vi "IMU Correction.vi"(9 "Heading Setpoint":dbl, 10 "theta":dbl) -> (3 "Difference":dbl)   [LabVIEW 2020]
panel:
  out "IMU Correction":T1(graph)
  in  "PID gains":T2={"proportional gain (Kp)"=4.0, "integral time (Ki)"=0.0, "derivative time (Kd)"=0.0} {"derivative time (Kd)" format="%.3f"; "integral time (Ki)" format="%.3f"; "proportional gain (Kp)" format="%.3f"}
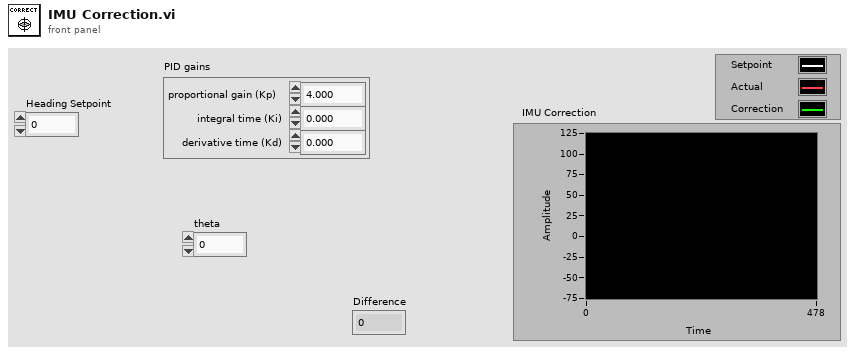
[diagram p1: front panel]
types:
  T1 = cluster{"Heading Setpoint":dbl, dbl, "output":dbl}
  T2 = cluster{"proportional gain (Kp)":dbl, "integral time (Ki)":dbl, "derivative time (Kd)":dbl}
  T3 = cluster{"Heading Setpoint":dbl, "theta":dbl, "output":dbl}
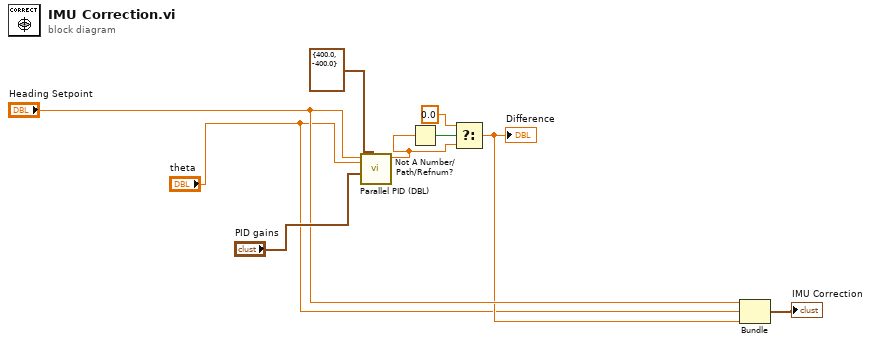
[diagram p0: block diagram]
diagram:
  n1 = call <vilib>:"Parallel PID (DBL).vi"("output range"=cluster{"output high":dbl, "output low":dbl} {"output high"=400.0, "output low"=-400.0}, "PID gains"="PID gains", "process variable"="theta", "setpoint"="Heading Setpoint") -> ("output"=w5:dbl)  [unwired: 4 in, 3 out]
  n2 = Not A Number/Path/Refnum?(number/path/refnum=w5) -> (NaN/Path/Refnum?=w9:bool)
  n3 = Select(t=0.0, s=w9, f=w5) -> (s? t:f=w2:dbl)
  "Difference" <- w2
  n4 = Bundle("Heading Setpoint"="Heading Setpoint", "theta"="theta", "output"=w2) -> (→"IMU Correction":T3)  [unwired: 1 in]
